vi "Add Node To Guarding.vi"(8 "error in":errorcluster, 9 "Timings":T1, 10 "Node ID":u8, 11 "Network Management in":refnum<class "Network Management.lvclass">) -> (0 "error out":errorcluster, 3 "Network Management out":refnum<class "Network Management.lvclass">)   [LabVIEW 2020, in "CANopen.lvlib" / "Network Management.lvlib" / "Network Management.lvclass"]
uses:
  Network Management.lvclass
  Network Management.lvclass/Network Management.ctl
  Node Guard Messages/Add Node Msg/Add Node Msg.lvclass
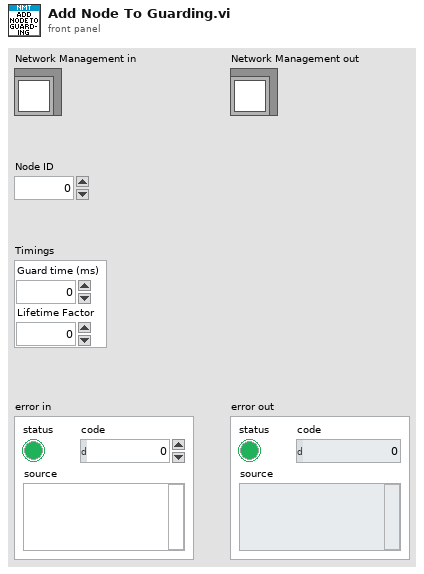
[diagram p1: front panel]
types:
  T1 = cluster{"Guard time (ms)":i32, "Lifetime Factor":u8}
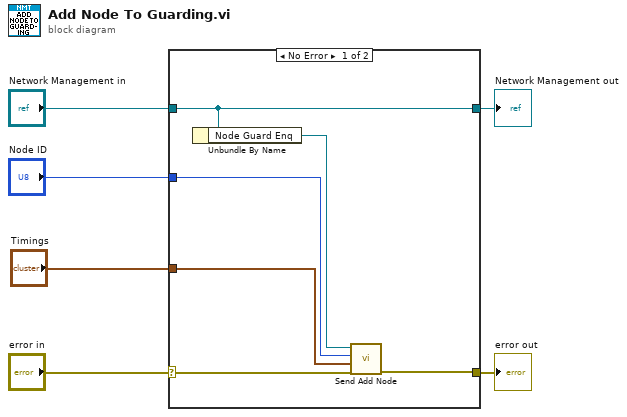
[diagram p0: block diagram]
diagram:
  n1 = case shown="No Error" "error in" {
    selector: "error in" -> [w11 w14]
    tunnel: [w10 w14] -> w3
    tunnel: [w12 w13] -> w5
    tunnel: "Network Management in" -> [w12 w13]
    tunnel: "Node ID" -> [w8 _]
    tunnel: "Timings" -> [w7 _]
    frame No Error {
      n2 = Unbundle By Name(w12) -> ("Node Guard Enq"=w9:refnum<class "Message Enqueuer.lvclass">)
      n3 = call "Send Add Node.vi"("error in (no error)"=w11, "Timings"=w7, "Node ID"=w8, "Message Enqueuer"=w9) -> ("error out"=w10:errorcluster)  [unwired: 6 in, 1 out]
    }
    frame Error {
    }
  }
  "Network Management out" <- w5
  "error out" <- w3
